vi "Read Original.vi"(11 "Sound Modification in":refnum<class "Sound Modification.lvclass">) -> (2 "Sound.lvclass":refnum<class "Sound.lvclass">, 3 "Sound Modification out":refnum<class "Sound Modification.lvclass">)   [LabVIEW 2010, in "Sound Modification.lvclass"]
uses:
  Sound Modification.lvclass
  Sound/Sound.lvclass
  Sound Modification.lvclass/Sound Modification.ctl
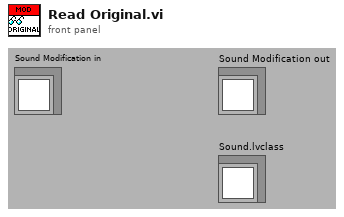
[diagram p1: front panel]
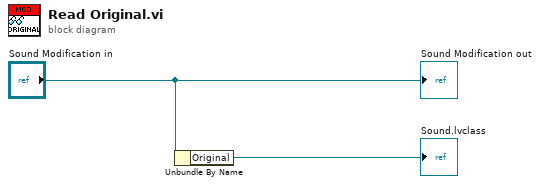
[diagram p0: block diagram]
diagram:
  n1 = Unbundle By Name("Sound Modification in") -> ("Original"=→"Sound.lvclass":refnum<class "Sound.lvclass">)
  "Sound Modification out" <- "Sound Modification in"
